vi "View_File.vi"(7 "File Selection":u16(ring), 8 "Error In":errorcluster, 11 "Data":T1={"Info Box"="", "MAC & Name Out"=[], "Default Gateway"="", "Drfiter IP Addresses"=[], "Network Map"="", "Drifter Selection"=0, "File Selection"=0, "Download File Path"=path "", "File Selection Strings"=[], "Sample Rate"=enum." 0.2", "Log While Charging"=enum." Yes"}) -> (0 "Error Out":errorcluster, 3 "File Contents":string)   [LabVIEW 2017]
uses:
  data.ctl
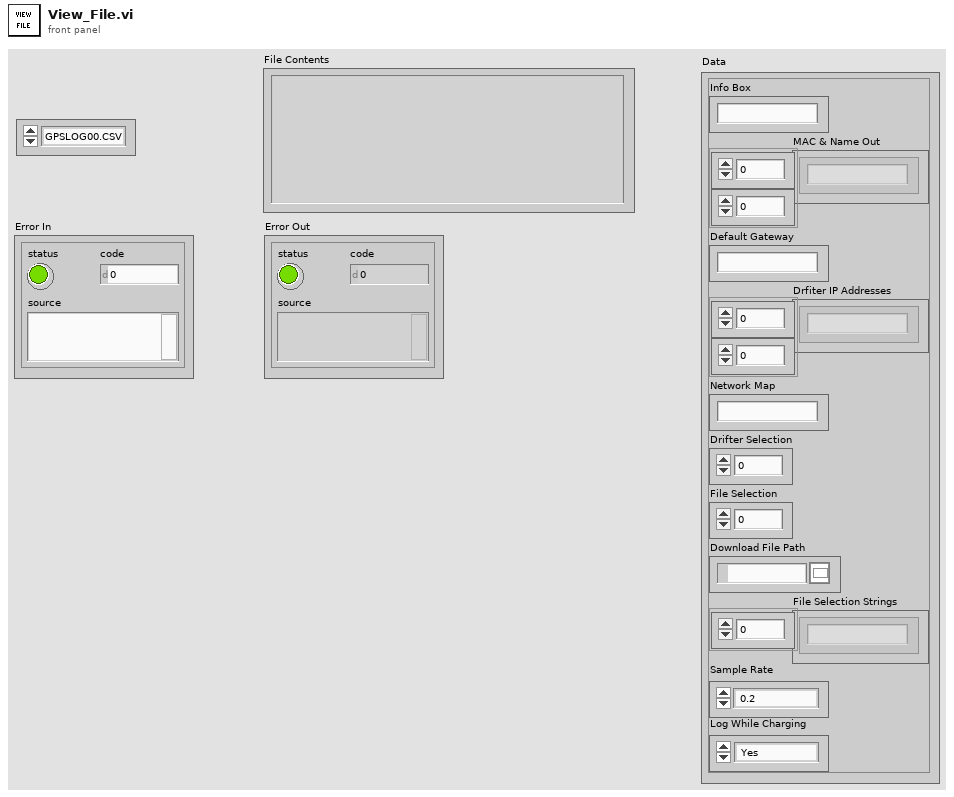
[diagram p1: front panel]
types:
  T1 = typedef "data.ctl" = cluster{"Info Box":string, "MAC & Name Out":string[][], "Default Gateway":string, "Drfiter IP Addresses":string[][], "Network Map":string, "Drifter Selection":i32, "File Selection":i32, "Download File Path":path, "File Selection Strings":string[], "Sample Rate":enum32{"No Selection", " 0.2", " 0.1", " 1", " 2", " 5", " 10"}, "Log While Charging":enum32{"No Selection", " Yes", " No"}}
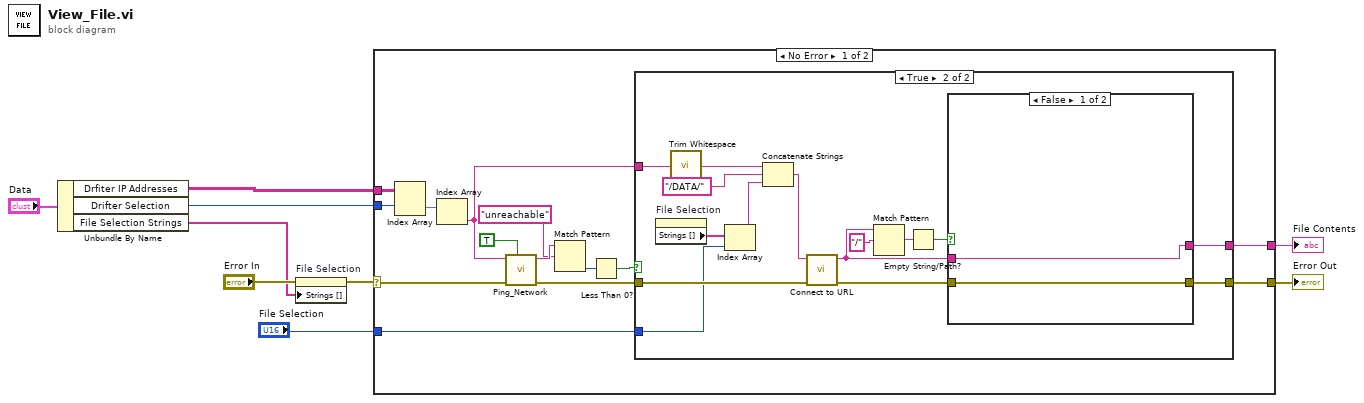
[diagram p0: block diagram]
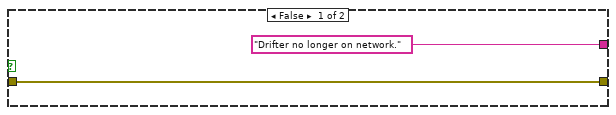
[diagram p2: hidden frame]
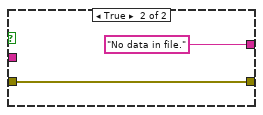
[diagram p3: hidden frame]
diagram:
  n1 = Unbundle By Name("Data") -> ("Drfiter IP Addresses"=w6:string[][], "Drifter Selection"=w5:i32, "File Selection Strings"=w1:string[])
  n2 = property on="File Selection" class="Ring (strict)"(error in="Error In", "Strings []"=w1) -> (error out=w2:errorcluster)  [unwired: 1 in, 1 out]
  n3 = case shown="No Error" w2 {
    selector: w2 -> [w12 w45]
    tunnel: [w23 w45] -> w8
    tunnel: w6 -> [w15 _]
    tunnel: [w13 _] -> w7
    tunnel: w5 -> [w11 _]
    tunnel: "File Selection" -> [w10 _]
    frame No Error {
      n4 = Index Array(array=w15, index (row)=w11) -> (element=w22:string[])  [unwired: 1 in]
      n5 = Index Array(array=w22) -> (element=w14:string)  [unwired: 1 in]
      n6 = call "Ping_Network.vi"("IP/Default Gateway (T/F)"=TRUE, "Error In"=w12, "Default Gateway/IP"=w14) -> ("Error Out"=w16:errorcluster, "Terminal Output"=w20:string)  [unwired: 7 in]
      n7 = Match Pattern(string=w20, regular expression="unreachable") -> (offset past match=w18:i32)  [unwired: 1 in, 3 out]
      n8 = Less Than 0?(x=w18) -> (x < 0?=w17:bool)
      n9 = case shown="True" w17 {
        tunnel: w16 -> [w25 w40]
        tunnel: [w25 w33] -> w23
        tunnel: w14 -> [_ w36]
        tunnel: ["Drifter no longer on network." ("Body") w35] -> w13
        tunnel: w10 -> [_ w31]
        frame False {
        }
        frame True {
          n10 = property on="File Selection" class="Ring (strict)"() -> ("Strings []"=w26:string[])  [unwired: 2 in, 2 out]
          n11 = call <vilib>:"Trim Whitespace.vi"("string"=w36) -> ("trimmed string"=w39:string)  [unwired: 1 in]
          n12 = Index Array(array=w26, index=w31) -> (element=w32:string)
          n13 = Concatenate Strings(w39, "/DATA/" ("string"), w32) -> (w37:string)
          n14 = call "Connect to URL.vi"("Error In"=w40, "URL"=w37) -> ("Error Out"=w34:errorcluster, "Body"=w28:string)  [unwired: 8 in]
          n15 = Match Pattern(string=w28, regular expression="/") -> (match substring=w27:string)  [unwired: 1 in, 3 out]
          n16 = Empty String/Path?(string/path=w27) -> (empty?=w30:bool)
          n17 = case shown="False" w30 {
            tunnel: [w41 "No data in file." ("Body")] -> w35
            tunnel: w28 -> [w41 _]
            tunnel: w34 -> [w42 w43]
            tunnel: [w42 w43] -> w33
            frame False {
            }
            frame True {
            }
          }
        }
      }
    }
    frame Error {
    }
  }
  "Error Out" <- w8
  "File Contents" <- w7
